vi "Close Helicopter Tasks.vi"(8 "Error In":errorcluster, 11 "Hellicopter Tasks Input 2":T1) -> (0 "Error Out":errorcluster)   [LabVIEW 2017]
uses:
  <vilib>/DAQmx/write.llb/DAQmx Write (Analog 1D DBL NChan 1Samp).vi
  <vilib>/DAQmx/miscellaneous.llb/DAQmx Fill In Error Info.vi
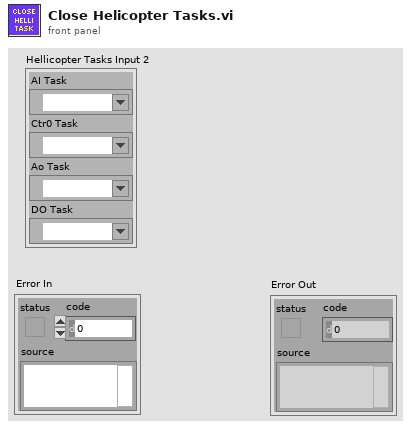
[diagram p1: front panel]
types:
  T1 = cluster{"AI Task":refnum<k21>, "Ctr0 Task":refnum<k21>, "Ao Task":refnum<k21>, "DO Task":refnum<k21>}
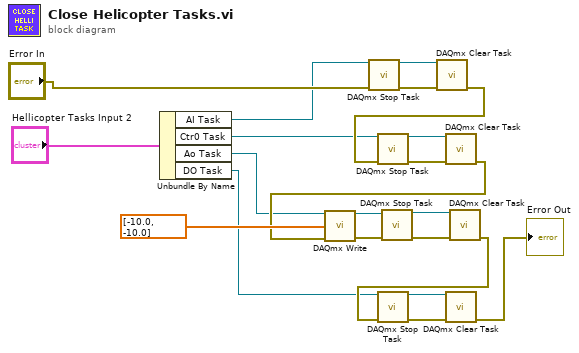
[diagram p0: block diagram]
diagram:
  n1 = Unbundle By Name("Hellicopter Tasks Input 2") -> ("AI Task"=w9:refnum<k21>, "Ctr0 Task"=w8:refnum<k21>, "Ao Task"=w7:refnum<k21>, "DO Task"=w2:refnum<k21>)
  n2 = call <vilib>:"DAQmx Stop Task.vi"("task/channels in"=w9, "error in"="Error In") -> ("task out"=w13:refnum<k21>, "error out"=w14:errorcluster)  [unwired: 12 in]
  n3 = call <vilib>:"DAQmx Clear Task.vi"("task in"=w13, "error in"=w14) -> ("error out"=w11:errorcluster)  [unwired: 13 in]
  n4 = call <vilib>:"DAQmx Stop Task.vi"("task/channels in"=w8, "error in"=w11) -> ("task out"=w16:refnum<k21>, "error out"=w15:errorcluster)  [unwired: 12 in]
  n5 = call <vilib>:"DAQmx Clear Task.vi"("task in"=w16, "error in"=w15) -> ("error out"=w12:errorcluster)  [unwired: 13 in]
  n6 = call-poly <vilib>:"DAQmx Write.vi"("task/channels in"=w7, "data"=dbl[] [-10.0, -10.0], "error in"=w12) -> ("task out"=w20:refnum<k21>, "error out"=w19:errorcluster)  [unwired: 10 in, 1 out]
  n7 = call <vilib>:"DAQmx Stop Task.vi"("task/channels in"=w20, "error in"=w19) -> ("task out"=w17:refnum<k21>, "error out"=w18:errorcluster)  [unwired: 12 in]
  n8 = call <vilib>:"DAQmx Clear Task.vi"("task in"=w17, "error in"=w18) -> ("error out"=w3:errorcluster)  [unwired: 13 in]
  n9 = call <vilib>:"DAQmx Stop Task.vi"("task/channels in"=w2, "error in"=w3) -> ("task out"=w1:refnum<k21>, "error out"=w5:errorcluster)  [unwired: 12 in]
  n10 = call <vilib>:"DAQmx Clear Task.vi"("task in"=w1, "error in"=w5) -> ("error out"=→"Error Out":errorcluster)  [unwired: 13 in]
